vi "mcl_connect.vi"(8 "error in (no error)":errorcluster, 11 "thorlabs_panel in":refnum<class "mcl_panel.lvclass">) -> (0 "error out":errorcluster, 3 "thorlabs_panel out":refnum<class "mcl_panel.lvclass">)   [LabVIEW 2015, in "mcl_panel.lvclass"]
uses:
  mcl_panel.lvclass
  mcl_piezo_class/mcl_piezo.lvclass
  mcl_panel.lvclass/mcl_panel.ctl
  UI/panel_class/panel.lvclass
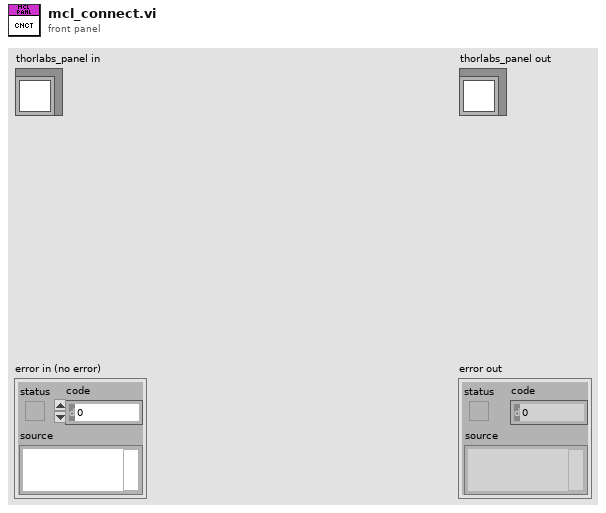
[diagram p1: front panel]
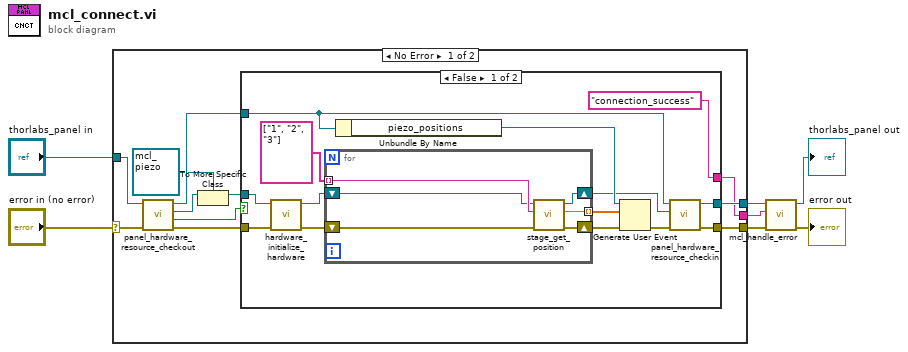
[diagram p0: block diagram]
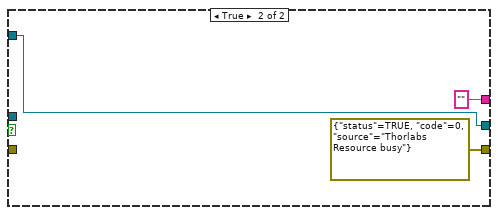
[diagram p2: hidden frame]
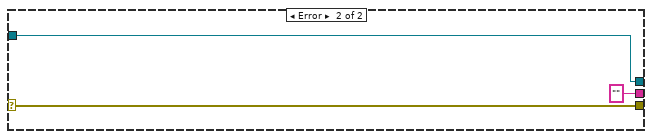
[diagram p3: hidden frame]
diagram:
  n1 = case shown="No Error" "error in (no error)" {
    selector: "error in (no error)" -> [w17 w44]
    tunnel: [w10 w44] -> w5
    tunnel: [w11 w43] -> w4
    tunnel: "thorlabs_panel in" -> [w18 w43]
    tunnel: [w8 "" ("event data")] -> w1
    frame No Error {
      n2 = call "panel_hardware_resource_checkout.vi"("error in (no error)"=w17, "panel in"=w18) -> ("error out"=w14:errorcluster, "timed out?"=w13:bool, "hardware.lvclass"=w16:refnum<class "hardware.lvclass">, "panel out"=w12:refnum<class "mcl_panel.lvclass">)  [unwired: 6 in]
      n3 = To More Specific Class(target class=refnum<class "mcl_piezo.lvclass"> refnum ("mcl_piezo.lvclass"), reference=w16) -> (specific class reference=w15:refnum<class "mcl_piezo.lvclass">)  [unwired: 1 in, 1 out]
      n4 = case shown="False" w13 {
        tunnel: w15 -> [w28 _]
        tunnel: w14 -> [w27 _]
        tunnel: w12 -> [w30 w40]
        tunnel: [w32 w40] -> w11
        tunnel: [w31 errorcluster {"status"=TRUE, "code"=0, "source"="Thorlabs Resource busy"} ("error out")] -> w10
        tunnel: ["connection_success" ("event data") "" ("event data")] -> w8
        frame False {
          n5 = call-dynamic "hardware_initialize_hardware.vi"("error in (no error)"=w27, "mcl_piezo in"=w28) -> ("error out"=w24:errorcluster, "mcl_piezo out"=w26:refnum<class "mcl_piezo.lvclass">)  [unwired: 8 in]
          n6 = for {
            tunnel: string[] ["1", "2", "3"] -> [w38] mode=indexing
            shift-right: [w35] -> w19
            shift-left: w26 -> [w36]
            tunnel: [w34] -> w23 mode=indexing
            shift-right: [w33] -> w22
            shift-left: w24 -> [w37]
            n7 = call-dynamic "stage_get_position.vi"("error in (no error)"=w37, "Stage Name"=w38, "mcl_piezo in"=w36) -> ("error out"=w33:errorcluster, "Position"=w34:dbl, "mcl_piezo out"=w35:refnum<class "mcl_piezo.lvclass">)  [unwired: 6 in]
          }
          n8 = Unbundle By Name(w30) -> ("piezo_positions"=w29:refnum<user-event>)
          n9 = Generate User Event(user event=w29, event data cluster=w23, error in=w22) -> (error out=w21:errorcluster)  [unwired: 1 in, 1 out]
          n10 = call "panel_hardware_resource_checkin.vi"("error in (no error)"=w21, "hardware.lvclass"=w19, "panel in"=w30) -> ("error out"=w31:errorcluster, "panel out"=w32:refnum<class "mcl_panel.lvclass">)  [unwired: 7 in]
        }
        frame True {
        }
      }
    }
    frame Error {
    }
  }
  n11 = call "mcl_handle_error.vi"("error in (no error)"=w5, "No Error String"=w1, "thorlabs_panel in"=w4) -> ("error out"=→"error out":errorcluster, "thorlabs_panel out"=→"thorlabs_panel out":refnum<class "mcl_panel.lvclass">)  [unwired: 7 in]
